vi "Rectangel RectangleLineOverlap.vi"(1 "bounds2":T1 {"height" format="%.2f"; "width" format="%.2f"; "y" format="%.2f"; "x" format="%.2f"}, 2 "bounds1":T1 {"height" format="%.2f"; "width" format="%.2f"; "y" format="%.2f"; "x" format="%.2f"}, 5 "error in (no error)":errorcluster) -> (15 "LineOverlap":bool, 19 "error out":errorcluster)   [LabVIEW 2020]
doc: "contains"
uses:
  <resource>/Framework/Providers/Open_GDS/UML/General/Rectangle/Rectangle Rectangle2D.ctl
  <resource>/Framework/Providers/Open_GDS/UML/General/Point/Point Point2D.ctl
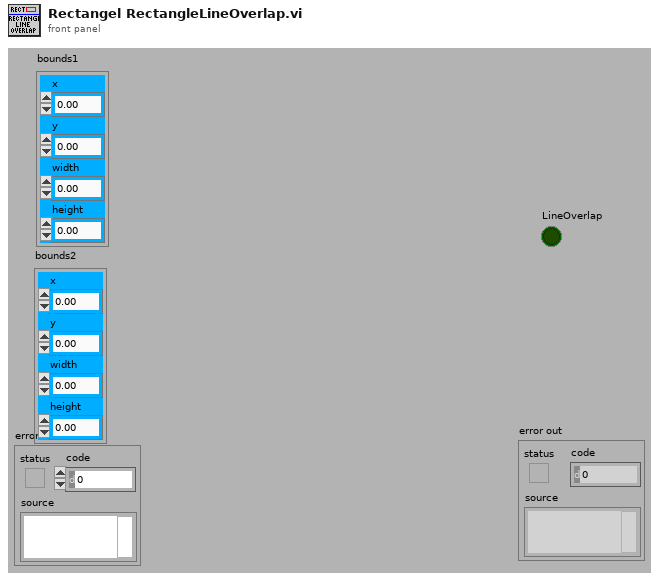
[diagram p1: front panel]
types:
  T1 = typedef "Rectangle Rectangle2D.ctl" = cluster{"x":dbl, "y":dbl, "width":dbl, "height":dbl}
  T2 = typedef "Point Point2D.ctl" = cluster{"x":dbl, "y":dbl}
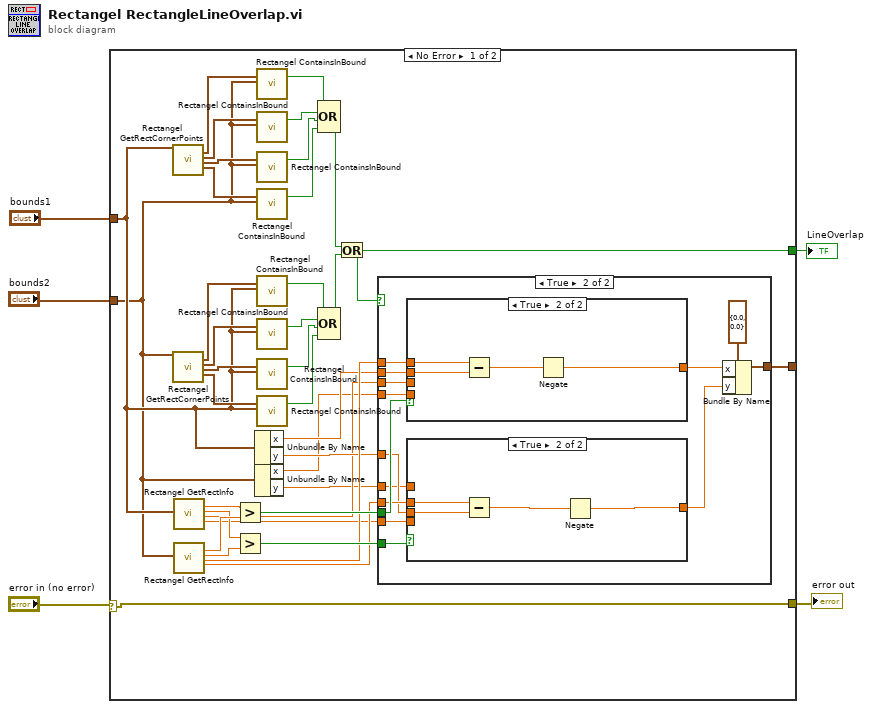
[diagram p0: block diagram]
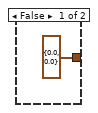
[diagram p2: hidden frame]
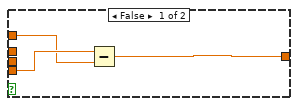
[diagram p3: hidden frame]
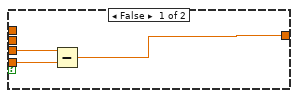
[diagram p4: hidden frame]
diagram:
  n1 = case shown="No Error" "error in (no error)" {
    selector: "error in (no error)" -> [w42 w72]
    tunnel: [w42 w72] -> w5
    tunnel: "bounds2" -> [w14 _]
    tunnel: "bounds1" -> [w15 _]
    tunnel: [w17 _] -> w1
    tunnel: [w16 _] -> _
    frame No Error {
      n2 = call <resource>:"Rectangel GetRectCornerPoints.vi"("bounds"=w15) -> ("X,Y"=w41:T2, "X+W,Y"=w39:T2, "X,Y+H"=w40:T2, "X+W,Y+H"=w38:T2)  [unwired: 1 in, 14 out]
      n3 = call <resource>:"Rectangel GetRectCornerPoints.vi"("bounds"=w14) -> ("X,Y"=w26:T2, "X+W,Y"=w28:T2, "X,Y+H"=w27:T2, "X+W,Y+H"=w29:T2)  [unwired: 1 in, 14 out]
      n4 = call <resource>:"Rectangel GetRectInfo.vi"("bounds"=w15) -> ("centerX"=w23:dbl, "centerY"=w21:dbl, "maxX"=w9:dbl, "maxY"=w7:dbl)  [unwired: 1 in, 14 out]
      n5 = call <resource>:"Rectangel GetRectInfo.vi"("bounds"=w14) -> ("centerX"=w22:dbl, "centerY"=w20:dbl, "maxX"=w13:dbl, "maxY"=w11:dbl)  [unwired: 1 in, 14 out]
      n6 = Greater?(x=w23, y=w22) -> (0:w19:bool)
      n7 = Greater?(x=w21, y=w20) -> (0:w18:bool)
      n8 = Unbundle By Name(w15) -> ("x"=w12:dbl, "y"=w10:dbl)
      n9 = Unbundle By Name(w14) -> ("x"=w8:dbl, "y"=w6:dbl)
      n10 = call <resource>:"Rectangel ContainsInBound.vi"("point2D"=w41, "bounds"=w14) -> ("contains"=w37:bool)  [unwired: 2 in, 15 out]
      n11 = call <resource>:"Rectangel ContainsInBound.vi"("point2D"=w39, "bounds"=w14) -> ("contains"=w36:bool)  [unwired: 2 in, 15 out]
      n12 = call <resource>:"Rectangel ContainsInBound.vi"("point2D"=w40, "bounds"=w14) -> ("contains"=w35:bool)  [unwired: 2 in, 15 out]
      n13 = call <resource>:"Rectangel ContainsInBound.vi"("point2D"=w38, "bounds"=w14) -> ("contains"=w34:bool)  [unwired: 2 in, 15 out]
      n14 = call <resource>:"Rectangel ContainsInBound.vi"("point2D"=w26, "bounds"=w15) -> ("contains"=w30:bool)  [unwired: 2 in, 15 out]
      n15 = call <resource>:"Rectangel ContainsInBound.vi"("point2D"=w28, "bounds"=w15) -> ("contains"=w31:bool)  [unwired: 2 in, 15 out]
      n16 = call <resource>:"Rectangel ContainsInBound.vi"("point2D"=w27, "bounds"=w15) -> ("contains"=w32:bool)  [unwired: 2 in, 15 out]
      n17 = call <resource>:"Rectangel ContainsInBound.vi"("point2D"=w29, "bounds"=w15) -> ("contains"=w33:bool)  [unwired: 2 in, 15 out]
      n18 = Compound Arithmetic op=OR(w37, w36, w35, w34) -> (w24:bool)
      n19 = Compound Arithmetic op=OR(w30, w31, w32, w33) -> (w25:bool)
      n20 = Or(x=w24, y=w25) -> (x .or. y?=w17:bool)
      n21 = case shown="True" w17 {
        tunnel: w19 -> [_ w55]
        tunnel: w18 -> [_ w44]
        tunnel: [T2 {"x"=0.0, "y"=0.0} ("translate1ToNotOverlap") w56] -> w16
        tunnel: w13 -> [_ w54]
        tunnel: w12 -> [_ w53]
        tunnel: w11 -> [_ w51]
        tunnel: w10 -> [_ w50]
        tunnel: w9 -> [_ w48]
        tunnel: w8 -> [_ w47]
        tunnel: w7 -> [_ w46]
        tunnel: w6 -> [_ w45]
        frame False {
        }
        frame True {
          n22 = case shown="True" w55 {
            tunnel: w54 -> [_ w71]
            tunnel: w53 -> [_ w70]
            tunnel: [w65 w68] -> w52
            tunnel: w48 -> [w67 _]
            tunnel: w47 -> [w66 _]
            frame False {
              n23 = Subtract(x=w67, y=w66) -> (x-y=w65:dbl)
            }
            frame True {
              n24 = Subtract(x=w71, y=w70) -> (x-y=w69:dbl)
              n25 = Negate(x=w69) -> (-x=w68:dbl)
            }
          }
          n26 = case shown="True" w44 {
            tunnel: w51 -> [_ w64]
            tunnel: w50 -> [_ w63]
            tunnel: [w58 w61] -> w49
            tunnel: w46 -> [w60 _]
            tunnel: w45 -> [w59 _]
            frame False {
              n27 = Subtract(x=w60, y=w59) -> (x-y=w58:dbl)
            }
            frame True {
              n28 = Subtract(x=w64, y=w63) -> (x-y=w62:dbl)
              n29 = Negate(x=w62) -> (-x=w61:dbl)
            }
          }
          n30 = Bundle By Name(cluster=T2 {"x"=0.0, "y"=0.0} ("translate1ToNotOverlap"), "x"=w52, "y"=w49) -> (w56:T2)
        }
      }
    }
    frame Error {
    }
  }
  "error out" <- w5
  "LineOverlap" <- w1
